vi "VI Tree.vi"   [LabVIEW 2016, in "Agilent N6700 Series.lvlib"]
doc: "This is the instrument driver for the Keysight/Agilent N6700 Series.\nThe VI Tree displays all the user-callable VIs of the instrument driver in an organized table."
uses:
  <instrlib>/Agilent N6700 Series/Agilent N6700 Series.lvlib
  <instrlib>/Agilent N6700 Series/Public/Configuration/Waveform/Configure Waveform (Exponential).vi
  <instrlib>/Agilent N6700 Series/Public/Configuration/Waveform/Sequence/Configure Sequence (Exponential).vi
panel:
  # "(c) 2004-2019  National Instruments.  ALL RIGHTS RESERVED."
  # "SEE DIAGRAM\nFOR VI TREE."
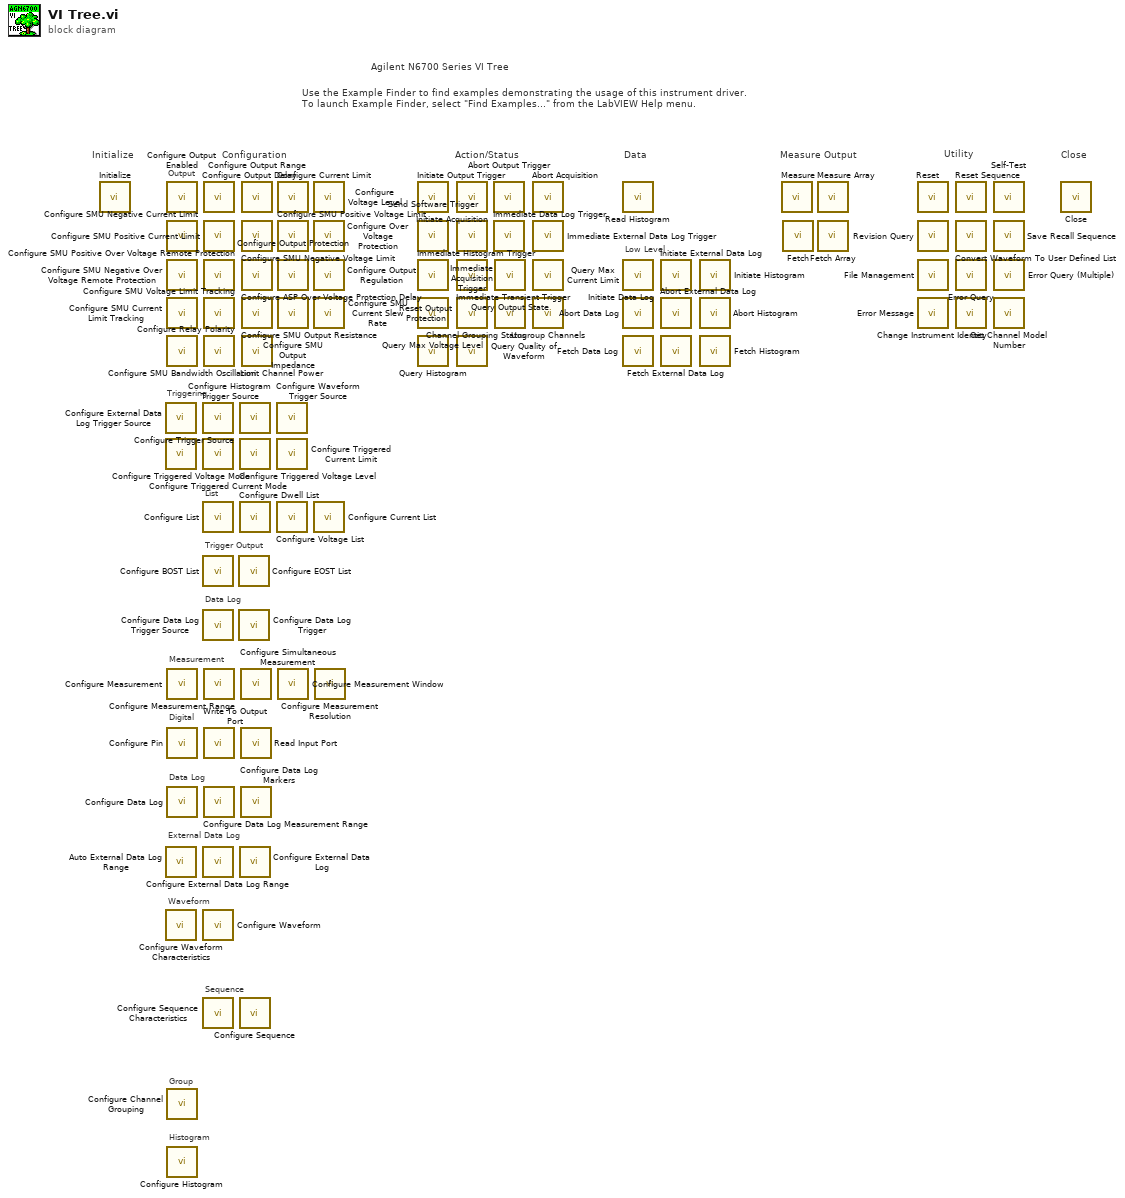
[diagram p0: block diagram]
diagram:
  # "External Data Log"
  # "Low Level"
  # "Sequence"
  # "Waveform"
  # "Data Log"
  # "Histogram"
  # "Data"
  # "Data Log"
  # "Measure Output"
  # "Agilent N6700 Series VI Tree"
  # "Use the Example Finder to find examples demonstrating the usage of this instrument driver.\nTo launch Example Finder, select \"Find Examples...\" from the LabVIEW Help menu."
  # "Configuration"
  # "Utility"
  # "Action/Status"
  # "Close"
  # "Initialize"
  # "Group"
  # "Digital"
  # "Measurement"
  # "Trigger Output"
  # "List"
  # "Triggering"
  # "Output"
  n1 = call <instrlib>:"Initialize.vi"() -> ()  [unwired: 14 in, 2 out]
  n2 = call <instrlib>:"Configure External Data Log Trigger Source.vi"() -> ()  [unwired: 10 in, 2 out]
  n3 = call <instrlib>:"Configure Triggered Voltage Mode.vi"() -> ()  [unwired: 10 in, 2 out]
  n4 = call <instrlib>:"Auto External Data Log Range.vi"() -> ()  [unwired: 10 in, 2 out]
  n5 = call <instrlib>:"Configure Waveform Characteristics.vi"() -> ()  [unwired: 10 in, 2 out]
  n6 = call <instrlib>:"Configure Output Enabled.vi"() -> ()  [unwired: 10 in, 2 out]
  n7 = call <instrlib>:"Configure SMU Negative Current Limit.vi"() -> ()  [unwired: 10 in, 2 out]
  n8 = call <instrlib>:"Configure SMU Negative Over Voltage Remote Protection.vi"() -> ()  [unwired: 10 in, 2 out]
  n9 = call <instrlib>:"Configure SMU Current Limit Tracking.vi"() -> ()  [unwired: 10 in, 2 out]
  n10 = call <instrlib>:"Configure SMU Bandwidth Oscillation.vi"() -> ()  [unwired: 10 in, 2 out]
  n11 = call <instrlib>:"Configure Measurement.vi"() -> ()  [unwired: 10 in, 2 out]
  n12 = call <instrlib>:"Configure Pin.vi"() -> ()  [unwired: 10 in, 2 out]
  n13 = call <instrlib>:"Configure Data Log.vi"() -> ()  [unwired: 10 in, 2 out]
  n14 = call <instrlib>:"Configure Channel Grouping.vi"() -> ()  [unwired: 10 in, 2 out]
  n15 = call <instrlib>:"Configure Histogram.vi"() -> ()  [unwired: 10 in, 2 out]
  n16 = call <instrlib>:"Configure Trigger Source.vi"() -> ()  [unwired: 10 in, 2 out]
  n17 = call <instrlib>:"Configure Triggered Current Mode.vi"() -> ()  [unwired: 10 in, 2 out]
  n18 = call <instrlib>:"Configure List.vi"() -> ()  [unwired: 10 in, 2 out]
  n19 = call <instrlib>:"Configure BOST List.vi"() -> ()  [unwired: 10 in, 2 out]
  n20 = call <instrlib>:"Configure Data Log Trigger Source.vi"() -> ()  [unwired: 10 in, 2 out]
  n21 = call <instrlib>:"Configure External Data Log Range.vi"() -> ()  [unwired: 10 in, 2 out]
  n22 = call-poly <instrlib>:"Configure Waveform.vi"() -> ()  [unwired: 14 in, 2 out]
  n23 = call <instrlib>:"Configure Sequence Characteristics.vi"() -> ()  [unwired: 14 in, 2 out]
  n24 = call <instrlib>:"Configure Output Delay.vi"() -> ()  [unwired: 10 in, 2 out]
  n25 = call <instrlib>:"Configure SMU Positive Current Limit.vi"() -> ()  [unwired: 10 in, 2 out]
  n26 = call <instrlib>:"Configure SMU Positive Over Voltage Remote Protection.vi"() -> ()  [unwired: 10 in, 2 out]
  n27 = call <instrlib>:"Configure SMU Voltage Limit Tracking.vi"() -> ()  [unwired: 10 in, 2 out]
  n28 = call <instrlib>:"Configure Relay Polarity.vi"() -> ()  [unwired: 10 in, 2 out]
  n29 = call <instrlib>:"Configure Measurement Range.vi"() -> ()  [unwired: 10 in, 2 out]
  n30 = call <instrlib>:"Write To Output Port.vi"() -> ()  [unwired: 10 in, 2 out]
  n31 = call <instrlib>:"Configure Data Log Measurement Range.vi"() -> ()  [unwired: 10 in, 2 out]
  n32 = call <instrlib>:"Configure EOST List.vi"() -> ()  [unwired: 10 in, 2 out]
  n33 = call <instrlib>:"Configure Data Log Trigger.vi"() -> ()  [unwired: 10 in, 2 out]
  n34 = call <instrlib>:"Configure Histogram Trigger Source.vi"() -> ()  [unwired: 10 in, 2 out]
  n35 = call <instrlib>:"Configure Triggered Voltage Level.vi"() -> ()  [unwired: 10 in, 2 out]
  n36 = call <instrlib>:"Configure Dwell List.vi"() -> ()  [unwired: 10 in, 2 out]
  n37 = call <instrlib>:"Configure External Data Log.vi"() -> ()  [unwired: 10 in, 2 out]
  n38 = call-poly <instrlib>:"Configure Sequence.vi"() -> ()  [unwired: 18 in, 2 out]
  n39 = call <instrlib>:"Configure Simultaneous Measurement.vi"() -> ()  [unwired: 10 in, 2 out]
  n40 = call <instrlib>:"Read Input Port.vi"() -> ()  [unwired: 9 in, 3 out]
  n41 = call <instrlib>:"Configure Data Log Markers.vi"() -> ()  [unwired: 10 in, 2 out]
  n42 = call <instrlib>:"Configure Output Range.vi"() -> ()  [unwired: 10 in, 2 out]
  n43 = call <instrlib>:"Configure SMU Negative Voltage Limit.vi"() -> ()  [unwired: 10 in, 2 out]
  n44 = call <instrlib>:"Configure ASP Over Voltage Protection Delay.vi"() -> ()  [unwired: 10 in, 2 out]
  n45 = call <instrlib>:"Configure SMU Output Resistance.vi"() -> ()  [unwired: 10 in, 2 out]
  n46 = call <instrlib>:"Limit Channel Power.vi"() -> ()  [unwired: 10 in, 2 out]
  n47 = call <instrlib>:"Configure Waveform Trigger Source.vi"() -> ()  [unwired: 10 in, 2 out]
  n48 = call <instrlib>:"Configure Triggered Current Limit.vi"() -> ()  [unwired: 10 in, 2 out]
  n49 = call <instrlib>:"Configure Voltage List.vi"() -> ()  [unwired: 10 in, 2 out]
  n50 = call <instrlib>:"Configure Current Limit.vi"() -> ()  [unwired: 10 in, 2 out]
  n51 = call <instrlib>:"Configure SMU Positive Voltage Limit.vi"() -> ()  [unwired: 10 in, 2 out]
  n52 = call <instrlib>:"Configure Output Protection.vi"() -> ()  [unwired: 10 in, 2 out]
  n53 = call <instrlib>:"Configure SMU Output Impedance.vi"() -> ()  [unwired: 10 in, 2 out]
  n54 = call <instrlib>:"Configure Measurement Window.vi"() -> ()  [unwired: 10 in, 2 out]
  n55 = call <instrlib>:"Configure Voltage Level.vi"() -> ()  [unwired: 10 in, 2 out]
  n56 = call <instrlib>:"Configure Over Voltage Protection.vi"() -> ()  [unwired: 10 in, 2 out]
  n57 = call <instrlib>:"Configure Output Regulation.vi"() -> ()  [unwired: 14 in, 2 out]
  n58 = call <instrlib>:"Configure SMU Current Slew Rate.vi"() -> ()  [unwired: 10 in, 2 out]
  n59 = call <instrlib>:"Configure Current List.vi"() -> ()  [unwired: 10 in, 2 out]
  n60 = call <instrlib>:"Configure Measurement Resolution.vi"() -> ()  [unwired: 10 in, 2 out]
  n61 = call <instrlib>:"Initiate Output Trigger.vi"() -> ()  [unwired: 10 in, 2 out]
  n62 = call <instrlib>:"Send Software Trigger.vi"() -> ()  [unwired: 10 in, 2 out]
  n63 = call <instrlib>:"Immediate Histogram Trigger.vi"() -> ()  [unwired: 10 in, 2 out]
  n64 = call <instrlib>:"Query Max Voltage Level.vi"() -> ()  [unwired: 9 in, 3 out]
  n65 = call <instrlib>:"Query Histogram.vi"() -> ()  [unwired: 11 in, 5 out]
  n66 = call <instrlib>:"Initiate Acquisition.vi"() -> ()  [unwired: 10 in, 2 out]
  n67 = call <instrlib>:"Immediate Acquisition Trigger.vi"() -> ()  [unwired: 10 in, 2 out]
  n68 = call <instrlib>:"Immediate Transient Trigger.vi"() -> ()  [unwired: 10 in, 2 out]
  n69 = call <instrlib>:"Reset Output Protection.vi"() -> ()  [unwired: 10 in, 2 out]
  n70 = call <instrlib>:"Query Quality of Waveform.vi"() -> ()  [unwired: 9 in, 3 out]
  n71 = call <instrlib>:"Abort Output Trigger.vi"() -> ()  [unwired: 10 in, 2 out]
  n72 = call <instrlib>:"Immediate Data Log Trigger.vi"() -> ()  [unwired: 10 in, 2 out]
  n73 = call <instrlib>:"Query Output State.vi"() -> ()  [unwired: 9 in, 3 out]
  n74 = call <instrlib>:"Channel Grouping Status.vi"() -> ()  [unwired: 9 in, 3 out]
  n75 = call <instrlib>:"Abort Acquisition.vi"() -> ()  [unwired: 10 in, 2 out]
  n76 = call <instrlib>:"Immediate External Data Log Trigger.vi"() -> ()  [unwired: 10 in, 2 out]
  n77 = call <instrlib>:"Query Max Current Limit.vi"() -> ()  [unwired: 9 in, 3 out]
  n78 = call <instrlib>:"Ungroup Channels.vi"() -> ()  [unwired: 10 in, 2 out]
  n79 = call <instrlib>:"Read Histogram.vi"() -> ()  [unwired: 9 in, 3 out]
  n80 = call <instrlib>:"Initiate Data Log.vi"() -> ()  [unwired: 10 in, 2 out]
  n81 = call <instrlib>:"Abort Data Log.vi"() -> ()  [unwired: 10 in, 2 out]
  n82 = call <instrlib>:"Fetch Data Log.vi"() -> ()  [unwired: 9 in, 3 out]
  n83 = call <instrlib>:"Initiate External Data Log.vi"() -> ()  [unwired: 10 in, 2 out]
  n84 = call <instrlib>:"Abort External Data Log.vi"() -> ()  [unwired: 10 in, 2 out]
  n85 = call <instrlib>:"Fetch External Data Log.vi"() -> ()  [unwired: 9 in, 3 out]
  n86 = call <instrlib>:"Initiate Histogram.vi"() -> ()  [unwired: 10 in, 2 out]
  n87 = call <instrlib>:"Abort Histogram.vi"() -> ()  [unwired: 10 in, 2 out]
  n88 = call <instrlib>:"Fetch Histogram.vi"() -> ()  [unwired: 9 in, 3 out]
  n89 = call <instrlib>:"Measure.vi"() -> ()  [unwired: 9 in, 3 out]
  n90 = call <instrlib>:"Fetch.vi"() -> ()  [unwired: 9 in, 3 out]
  n91 = call <instrlib>:"Measure Array.vi"() -> ()  [unwired: 8 in, 4 out]
  n92 = call <instrlib>:"Fetch Array.vi"() -> ()  [unwired: 8 in, 4 out]
  n93 = call <instrlib>:"Reset.vi"() -> ()  [unwired: 14 in, 2 out]
  n94 = call <instrlib>:"Revision Query.vi"() -> ()  [unwired: 12 in, 4 out]
  n95 = call <instrlib>:"File Management.vi"() -> ()  [unwired: 10 in, 2 out]
  n96 = call <instrlib>:"Error Message.vi"() -> ()  [unwired: 11 in, 5 out]
  n97 = call <instrlib>:"Reset Sequence.vi"() -> ()  [unwired: 10 in, 2 out]
  n98 = call <instrlib>:"Convert Waveform To User Defined List.vi"() -> ()  [unwired: 10 in, 2 out]
  n99 = call <instrlib>:"Error Query.vi"() -> ()  [unwired: 12 in, 4 out]
  n100 = call <instrlib>:"Change Instrument Identity.vi"() -> ()  [unwired: 10 in, 2 out]
  n101 = call <instrlib>:"Self-Test.vi"() -> ()  [unwired: 12 in, 4 out]
  n102 = call <instrlib>:"Save Recall Sequence.vi"() -> ()  [unwired: 10 in, 2 out]
  n103 = call <instrlib>:"Error Query (Multiple).vi"() -> ()  [unwired: 12 in, 4 out]
  n104 = call <instrlib>:"Get Channel Model Number.vi"() -> ()  [unwired: 9 in, 3 out]
  n105 = call <instrlib>:"Close.vi"() -> ()  [unwired: 15 in, 1 out]
